vi "PCSMain.Free PHELIX Switch Instances.vi"(1 "DB Entries":cluster{"Object Name":string, "Class":string}[](array[cluster])) -> (0 "Free Switch GUI elements":cluster{"Object Name":string, "Class":string}[](array[cluster]))   [LabVIEW 2014, in "PCSMain.lvlib"]
doc: "This VI acts as a filter: From the input data base entries, it gives out all which are belonging to the classes PH_Switch, PH_Sixpack_Switch except those named inside the block diagram. This VI is meant to be used in MainGUIs."
uses:
  PCSMain.lvlib
  PH_Beamline/PH_Beamline.Switch GUI Instances.ctl
  PH_Beamline/PH_Beamline.Switch+6P Instances.ctl
  PH_Beamline/PH_Beamline.6P Switch Instances.ctl
  PH_Beamline/PH_Beamline.Switch Instances.ctl
  Z6_Beamline/Z6_Beamline.6P Switch Instances.ctl
  Z6_Beamline/Z6_Beamline.Switch Instances.ctl
  Z6_Beamline/Z6_Beamline.Switch+6P Instances.ctl
  PH_Beamline/PH_Beamline.lvlib
  Z6_Beamline/Z6_Beamline.lvlib
panel:
  in  "Z6 Switch and 6P Instances":T1="N/A"
  in  "Z6 Switch Instances":T2="Shutter_Exp4"
  in  "Z6 6P Switch Instances":T3="N/A"
  in  "Switch Instances":T4="MA01_CH1"
  in  "6P Switch Instances":T5="MA01_CH1"
  in  "Switch and 6P Instances":T6="BL_Position_MM5::MA_MM5_6PGUI"
  in  "Switch GUI Instances":T7="Shutter_Exp_Laserbay_Interlock"
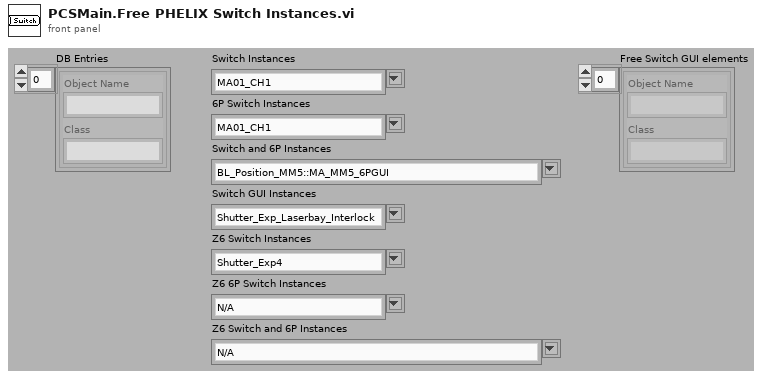
[diagram p1: front panel]
types:
  T1 = typedef "Z6_Beamline.lvlib/Z6_Beamline.Switch+6P Instances.ctl" = string
  T2 = typedef "Z6_Beamline.lvlib/Z6_Beamline.Switch Instances.ctl" = string
  T3 = typedef "Z6_Beamline.lvlib/Z6_Beamline.6P Switch Instances.ctl" = string
  T4 = typedef "PH_Beamline.lvlib/PH_Beamline.Switch Instances.ctl" = string
  T5 = typedef "PH_Beamline.lvlib/PH_Beamline.6P Switch Instances.ctl" = string
  T6 = typedef "PH_Beamline.lvlib/PH_Beamline.Switch+6P Instances.ctl" = string
  T7 = typedef "PH_Beamline.lvlib/PH_Beamline.Switch GUI Instances.ctl" = string
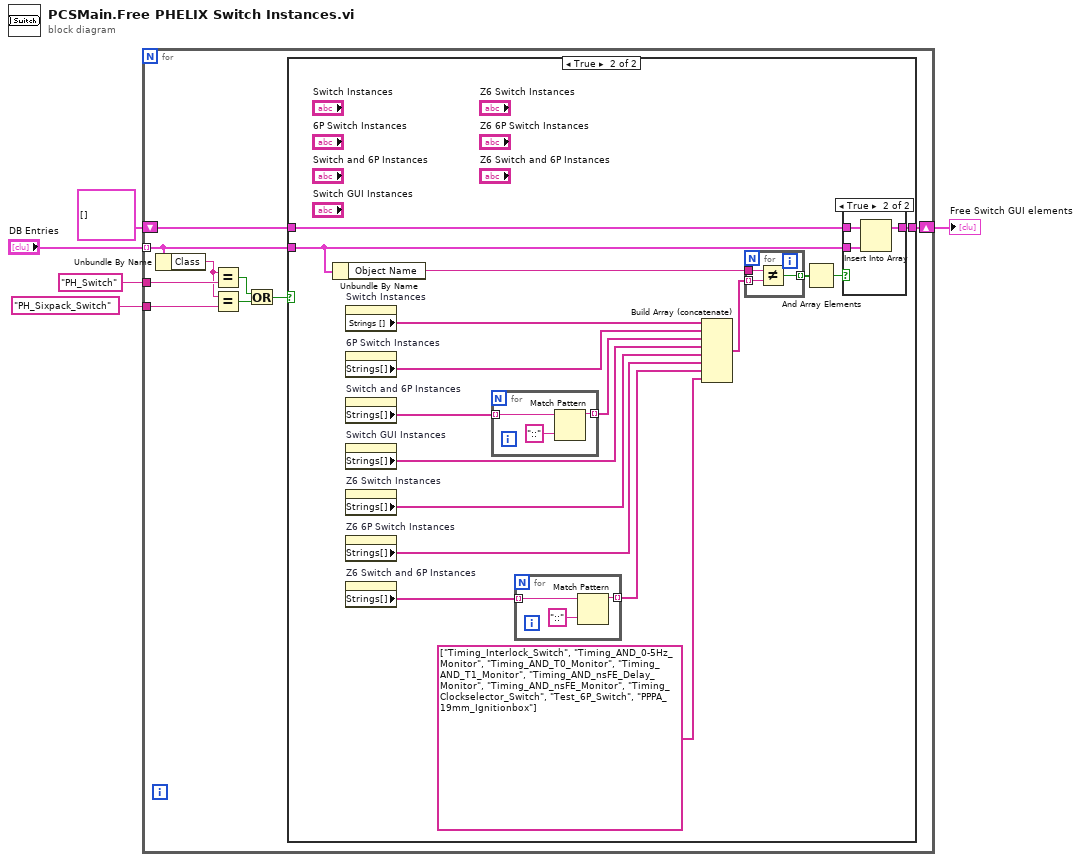
[diagram p0: block diagram]
diagram:
  n1 = for {
    tunnel: "PH_Switch" ("Class") -> [w14]
    tunnel: "DB Entries" -> [w13] mode=indexing
    shift-right: [w12] -> w1
    shift-left: cluster{"Object Name":string, "Class":string}[] [] -> [w11]
    tunnel: "PH_Sixpack_Switch" ("Class") -> [w9]
    n2 = Unbundle By Name(w13) -> ("Class"=w10:string)
    n3 = Equal?(x=w10, y=w14) -> (x = y?=w7:bool)
    n4 = Equal?(x=w10, y=w9) -> (x = y?=w8:bool)
    n5 = Or(x=w7, y=w8) -> (x .or. y?=w6:bool)
    n6 = case shown="True" w6 {
      tunnel: w13 -> [_ w30]
      tunnel: [w15 w32] -> w12
      tunnel: w11 -> [w15 w31]
      frame False {
      }
      frame True {
        n7 = Unbundle By Name(w30) -> ("Object Name"=w29:string)
        n8 = property on="Switch Instances" class="CmbBox (strict)"() -> ("Strings []"=w26:string[])  [unwired: 2 in, 2 out]
        n9 = property on="6P Switch Instances" class="CmbBox (strict)"() -> ("Strings[]"=w24:string[])  [unwired: 2 in, 2 out]
        n10 = property on="Switch and 6P Instances" class="CmbBox (strict)"() -> ("Strings[]"=w23:string[])  [unwired: 2 in, 2 out]
        n11 = property on="Switch GUI Instances" class="CmbBox (strict)"() -> ("Strings[]"=w21:string[])  [unwired: 2 in, 2 out]
        n12 = property on="Z6 Switch Instances" class="CmbBox (strict)"() -> ("Strings[]"=w18:string[])  [unwired: 2 in, 2 out]
        n13 = property on="Z6 6P Switch Instances" class="CmbBox (strict)"() -> ("Strings[]"=w17:string[])  [unwired: 2 in, 2 out]
        n14 = property on="Z6 Switch and 6P Instances" class="CmbBox (strict)"() -> ("Strings[]"=w19:string[])  [unwired: 2 in, 2 out]
        n15 = for {
          tunnel: w23 -> [w38] mode=indexing
          tunnel: [w36] -> w22 mode=indexing
          n16 = Match Pattern(string=w38, regular expression="::") -> (before substring=w36:string)  [unwired: 1 in, 3 out]
        }
        n17 = for {
          tunnel: w19 -> [w35] mode=indexing
          tunnel: [w33] -> w16 mode=indexing
          n18 = Match Pattern(string=w35, regular expression="::") -> (before substring=w33:string)  [unwired: 1 in, 3 out]
        }
        n19 = Build Array (concatenate)(w26, w24, w22, w21, w18, w17, w16, string[] ["Timing_Interlock_Switch", "Timing_AND_0-5Hz_Monitor", "Timing_AND_T0_Monitor", "Timing_AND_T1_Monitor", "Timing_AND_nsFE_Delay_Monitor", "Timing_AND_nsFE_Monitor", "Timing_Clockselector_Switch", "Test_6P_Switch", "PPPA_19mm_Ignitionbox"]) -> (w25:string[])
        n20 = for {
          tunnel: w29 -> [w44]
          tunnel: w25 -> [w43] mode=indexing
          tunnel: [w45] -> w28 mode=indexing
          n21 = Not Equal?(x=w44, y=w43) -> (x != y?=w45:bool)
        }
        n22 = And Array Elements(Boolean array=w28) -> (logical AND=w27:bool)
        n23 = case shown="True" w27 {
          tunnel: [w39 w42] -> w32
          tunnel: w31 -> [w39 w41]
          tunnel: w30 -> [_ w40]
          frame False {
          }
          frame True {
            n24 = Insert Into Array(array=w41, new element=w40) -> (w42:cluster{"Object Name":string, "Class":string}[])  [unwired: 1 in]
          }
        }
      }
    }
  }
  "Free Switch GUI elements" <- w1
